vi "SPC_read_data_block.vi"(5 "page":i32, 6 "Data Buffer":u16[](array[numeric]), 7 "to":i16, 8 "Error In":errorcluster, 9 "block":i32, 10 "Module No":i16, 11 "DLL Path":path) -> (0 "Error Out":errorcluster, 2 "Module No":i16, 3 "DLL Path":path, 4 "Data":u16[](array[numeric]))   [LabVIEW 2019]
doc: "B&H suggests using the VI <b>SPC_read_block.vi</b> instead.\n\nThe procedure reads data from a block of the SPC memory (on module 'mod_no') defined by the parameters 'block' and 'page' to the buffer 'data'. The procedure is used to read measurement results from the SPC memory.\nThe function performs a data reduction by averaging a specified number of data points into one result value. \nThe parameter 'reduction_factor' defines the number of points that are averaged. \nThe value of 'reduction_factor' must be a power of 2. The number of values stored in 'data'(named below no_of_points) is equal to block length divided by reduction_factor.\nThe parameters 'from' and 'to' define the address range inside the buffer 'data' i.e. refer to the (compressed) destination data. 'from' and 'to' must be in the range from 0 to no_of_points-1. \nThe parameter 'to' must be greater than or equal to the parameter 'from'.\nThe range of the parameters 'block' and 'page' depends on the actual configuration of the SPC memory (see SPC_configure_memory).\nThe assumption is done that frames_per_page is equal 1 ( page = frame ) (see 'Memory Configuration).\nTo provide correct access to the SPC memory it is required that the function SPC_configure_memory be used ( in normal operation modes) before the first call of SPC_read_data_block. \nThis function also delivers the required information about the block/page structure of the SPC memory:\nlong max_block_no total number of blocks (=curves) in the memory ( memory bank for the SPC- 6x0/13x/15x/160)\nlong blocks_per_frame Number of blocks (=curves) per frame\nlong frames_per_page Number of frames per page\nlong maxpage max number of pages to use in a measurement\nlong block_length Number of 16-bits words per one block (curve)\nPlease make sure that the buffer 'data' be allocated with enough memory for no_of_points.\n<b>Note:</b> This VI is set to execute as preallocated clone to improve performance when run in parallel loops for multi module setups. \n\ninfo@becker-hickl.com"
panel:
  in  "reduction_factor":i16=1 min=1 max=2048 step=1
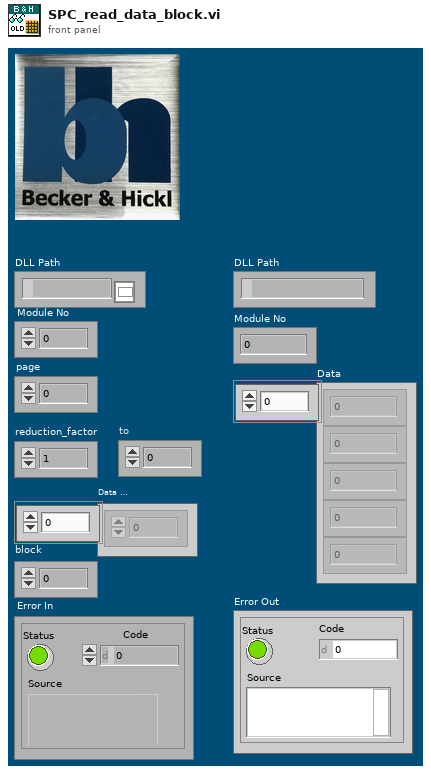
[diagram p1: front panel]
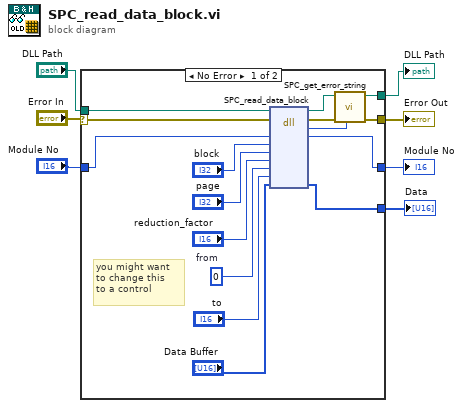
[diagram p0: block diagram]
diagram:
  n1 = case shown="No Error" "Error In" {
    selector: "Error In" -> [w23 w26]
    tunnel: [w18 w25] -> w7
    tunnel: [w17 w26] -> w6
    tunnel: "DLL Path" -> [w22 w25]
    tunnel: "Module No" -> [w13 w24]
    tunnel: [w12 w24] -> w2
    tunnel: [w9 _] -> w1
    frame No Error {
      w15 = i16 0  # from
      # "you might want \nto change this \nto a control"
      n2 = dll-call lib="C:/Program Files (x86)/BH/SPCM/DLL/spcm64.dll" fn="SPC_read_data_block"(path in=w22, error in=w23, "mod_no"=w13, "block"="block", "page"="page", "reduction_factor"="reduction_factor", "from"=w15, "to"="to", "data"="Data Buffer") -> (path out=w19:path, error out=w20:errorcluster, "return type"=w21:i16, "mod_no"=w12:i16, "data"=w9:u16[])  [unwired: 6 in]
      n3 = call "SPC_get_error_string.vi"("ErrorID"=w21, "Error In"=w20, "DLL Path"=w19) -> ("Error Out"=w17:errorcluster, "DLL Path"=w18:path)  [unwired: 6 in, 1 out]
    }
    frame Error {
    }
  }
  "DLL Path" <- w7
  "Error Out" <- w6
  "Module No" <- w2
  "Data" <- w1
